vi "Handle Notification.vi"(8 "error in (no error)":errorcluster, 9 "Payload":string, 10 "Notification Type":string, 11 "Spectrogram in":refnum<class "Spectrogram.lvclass">) -> (0 "error out":errorcluster, 3 "Spectrogram out":refnum<class "Spectrogram.lvclass">)   [LabVIEW 2023, in "Spectrogram.lvlib" / "Spectrogram.lvclass"]
uses:
  Spectrogram.lvclass
  Spectrogram.lvclass/Spectrogram.ctl
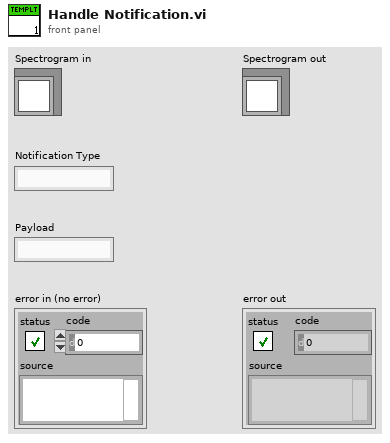
[diagram p1: front panel]
types:
  T1 = typedef "Spectrogram.lvlib/Spectrogram.lvclass/Spectrogram Data.ctl" = cluster{"Show Spectrogram Window":bool, "Show Spectrogram Window Button Clicked":bool, "Spectrogram VI Ref":refnum<vi>, "Extension":u16, "Time steps":i32, "Frequency bins":i32, "Type":i32, "Length":i32, "Color Table":u16}
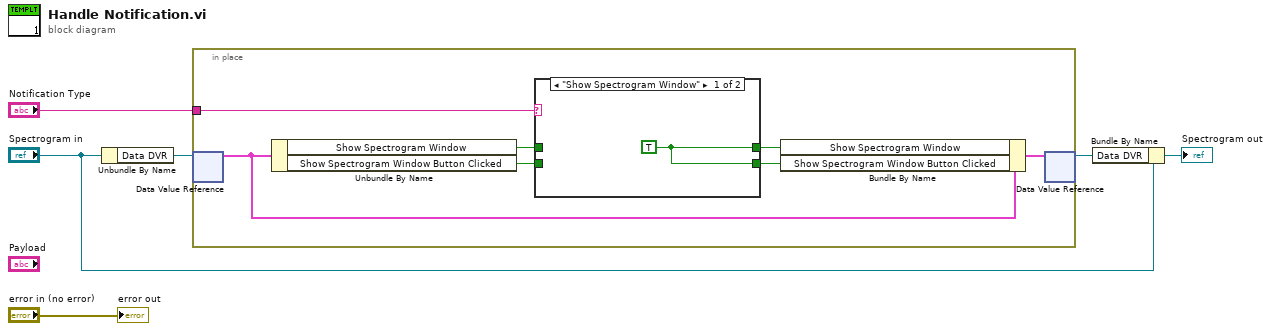
[diagram p0: block diagram]
diagram:
  n1 = Unbundle By Name("Spectrogram in") -> ("Data DVR"=w4:refnum<data-value>)
  n2 = in-place {
    in-place-border: "Notification Type" -> [w13]
    n3 = in-place-dvr #1(w4) -> (w10:T1)  [unwired: 1 out]
    n4 = Unbundle By Name(w10) -> ("Show Spectrogram Window"=w12:bool, "Show Spectrogram Window Button Clicked"=w11:bool)
    n5 = case shown="\"Show Spectrogram Window\"" w13 {
      tunnel: [w14 w16] -> w9
      tunnel: w12 -> [_ w16]
      tunnel: w11 -> [_ w15]
      tunnel: [w14 w15] -> w8
      frame "Show Spectrogram Window" {
        w14 = TRUE
      }
      frame Default {
      }
    }
    n6 = Bundle By Name(cluster=w10, "Show Spectrogram Window"=w9, "Show Spectrogram Window Button Clicked"=w8) -> (w7:T1)
    n7 = in-place-dvr #1(w7) -> (w2:refnum<data-value>)  [unwired: 1 out]
  }
  n8 = Bundle By Name(cluster="Spectrogram in", "Data DVR"=w2) -> (→"Spectrogram out":refnum<class "Spectrogram.lvclass">)
  "error out" <- "error in (no error)"
